vi "FPGA.vi"() -> ()   [LabVIEW 2014]
uses:
  SPI v2/ADXL345 Output.ctl
  <userlib>/_NI SPI IP/FPGA/Controllers/Public/Transfer Settings.ctl
  SPI v2/ADXL345 SPI Statechart.lvsc/Outputs.ctl
  <vilib>/Platform/TimedLoop/XDataNode/timing_clust.ctl
  <vilib>/Platform/TimedLoop/XDataNode/nitl_modes.ctl
  <vilib>/Platform/TimedLoop/XDataNode/wakeup.ctl
  <userlib>/_NI SPI IP/FPGA/Controllers/Public/Spi Master Inputs.ctl
  SPI v2/ADXL345 SPI Statechart.lvsc/Inputs.ctl
  <vilib>/rvi/Emulation/niFpgaGetClockAttributes.vi
  <vilib>/rvi/Emulation/niFpgaSctlEmulationGetInTimedLoop.vi
  <vilib>/rvi/Emulation/niFpgaEmulationReportErrorSimple.vi
  <vilib>/rvi/eio/common/nirviEmuTemplateMethod_errors.vi
  FPGA Globals.vi
  <vilib>/rvi/Emulation/niFpgaCriticalErrorInLSC.vi
  <vilib>/rvi/Emulation/niFpgaProcessEmulError.vi
  SPI v2/ADXL345 SPI Statechart.lvsc/CompanionDiagram.vi/7/SC Main.vi
  <vilib>/eio/EIONode/EIONode.xnode
  <vilib>/rvi/Analysis/measure/butterworth/XNode/niFpgaButterworthFilter.xnode
  <vilib>/Platform/TimedLoop/XDataNode/XDataNode.xnode
  SPI v2/ADXL345 SPI Statechart.lvsc/Trigger.ctl
  <vilib>/Statechart/Infrastructure/RTStatechart/RunTime SCN.xnode
  SPI v2/ADXL345 SPI Statechart.lvsc
  <vilib>/Platform/TimedLoop/XDataNode/XDNodeRunTimeDep.lvlib
  <userlib>/_NI SPI IP/FPGA/Controllers/NI SPI IP FPGA.lvlib
panel:
  in  "bDCDCDisable":bool
  in  "bLapBeaconPickupEnable":bool
  in  "bWheelSpeedsEnable":bool
  in  "bAccumulatorFansEnable":bool
  out "bLapBeaconPickup":bool
  out "tLapDelta":u32
  in  "bResetFastestLap":bool
  out "tFastestLap":u32
  in  "tLapReference":u32
  in  "bWheelFRFail":bool
  in  "bWheelFLFail":bool
  out "ADXL345 Output":T1
  out "rSlipFR":fxp<+/-,12,1>
  out "rSlipFL":fxp<+/-,12,1>
  out "rSlipRR":fxp<+/-,12,1>
  out "rSlipRL":fxp<+/-,12,1>
  out "sLap":fxp<+,32,12>
  out "vCar":fxp<+/-,33,19>
  out "vAxleF":fxp<+/-,33,19>
  in  "bAccel":bool
  out "vWheelHighest":fxp<+/-,32,18>
  out "vWheelLowest":fxp<+/-,32,18>
  out "vWheelFL":fxp<+/-,32,18>
  out "vWheelFR":fxp<+/-,32,18>
  out "vWheelRL":fxp<+/-,32,18>
  out "vWheelRR":fxp<+/-,32,18>
  in  "Tire Diameter(m)":fxp<+,16,1>
  out "nWheelRR":fxp<+/-,29,16>
  out "nWheelRL":fxp<+/-,29,16>
  out "nWheelFR":fxp<+/-,29,16>
  out "nWheelFL":fxp<+/-,29,16>
  out "NLap":u8
  in  "bResetNLap":bool
  out "aSteerWheel":fxp<+/-,22,10>=124.904541015625
  in  "VSteerWheelMiddle":fxp<+/-,26,5>=0.34827280044555664
  out "bBrakeFOK":bool
  out "bBrakeROK":bool
  out "bLowCurrentOK":bool
  out "bHighCurrentOK":bool
  out "pBrakeF":fxp<+,26,13>
  out "pBrakeR":fxp<+,26,13>
  out "ILowCurrent":fxp<+/-,24,15>=4.353515625
  out "IHighCurrent":fxp<+/-,24,15>=-20.724609375
  out "VShockFL":fxp<+/-,24,5>=0.3892974853515625
  out "VShockFR":fxp<+/-,24,5>=0.3425788879394531
  out "VShockRL":fxp<+/-,24,5>=0.3444976806640625
  out "VShockRR":fxp<+/-,24,5>=0.3793773651123047
  in  "bBrakeLight":bool=TRUE
  out "tWheelFLPeriod":u32
  out "tWheelFRPeriod":u32
  out "tWheelRRPeriod":u32
  out "tWheelRLPeriod":u32
  out "bWheelFLStopped":bool=TRUE
  out "bWheelFRStopped":bool=TRUE
  out "bWheelRLStopped":bool=TRUE
  out "bWheelRRStopped":bool=TRUE
  out "VBrakePressureF":fxp<+/-,24,5>=0.4808177947998047
  out "VBrakePressureR":fxp<+/-,24,5>=0.4820976257324219
  out "bWheelFL":bool
  out "bWheelFR":bool
  out "bWheelRR":bool
  out "bWheelRL":bool
  out "V5VSupply":fxp<+/-,24,5>
  in  "tLapMin":u32=15000
  out "tLastLap":u32
  out "bNewLap":bool
  out "tCurrentLap":u32
  in  "bMotorControllerEnable":bool
  out "bTSMSOutStatus":bool
  in  "bSBRIOOK1":bool
  in  "bSBRIOOK2":bool
  out "bBSPDOK":bool
  out "bIMDOK":bool
  out "bBMSOK":bool
  in  "bPosAIREnable":bool
  out "bTSMSInStatus":bool
  in  "bRTDSEnable":bool
  in  "bCoolantPumpEnable":bool
  in  "rTPS1Min":fxp<+,16,4>=0.41015625
  in  "rTPS1Max":fxp<+,16,4>=0.6201171875
  in  "rTPS2Min":fxp<+,16,4>=0.489990234375
  in  "rTPS2Max":fxp<+,16,4>=0.27001953125
  out "rTPS1":fxp<+/-,31,22>
  out "VTPS1":fxp<+/-,24,5>=3.619058609008789
  out "rTPS2":fxp<+/-,31,22>
  out "VTPS2":fxp<+/-,24,5>=1.0001773834228516
  out "rThrottle":fxp<+/-,33,22>
  out "bTPSInRange":bool
  out "bTPSConsistent":bool
  out "rTPS1Unscaled":fxp<+/-,16,1>
  out "rTPS2Unscaled":fxp<+/-,16,1>
  out "TSBRIO":fxp<+,19,8>=27.25 format="%.10g"
  out "bFPGALED":bool
  out "VsbRIOSupply":fxp<+/-,25,6>=13.101043701171875
  in  "VSupplyOffset":fxp<+,12,4>=8.890625
  in  "stop":bool
  out "Tick Count(mSec)":u32
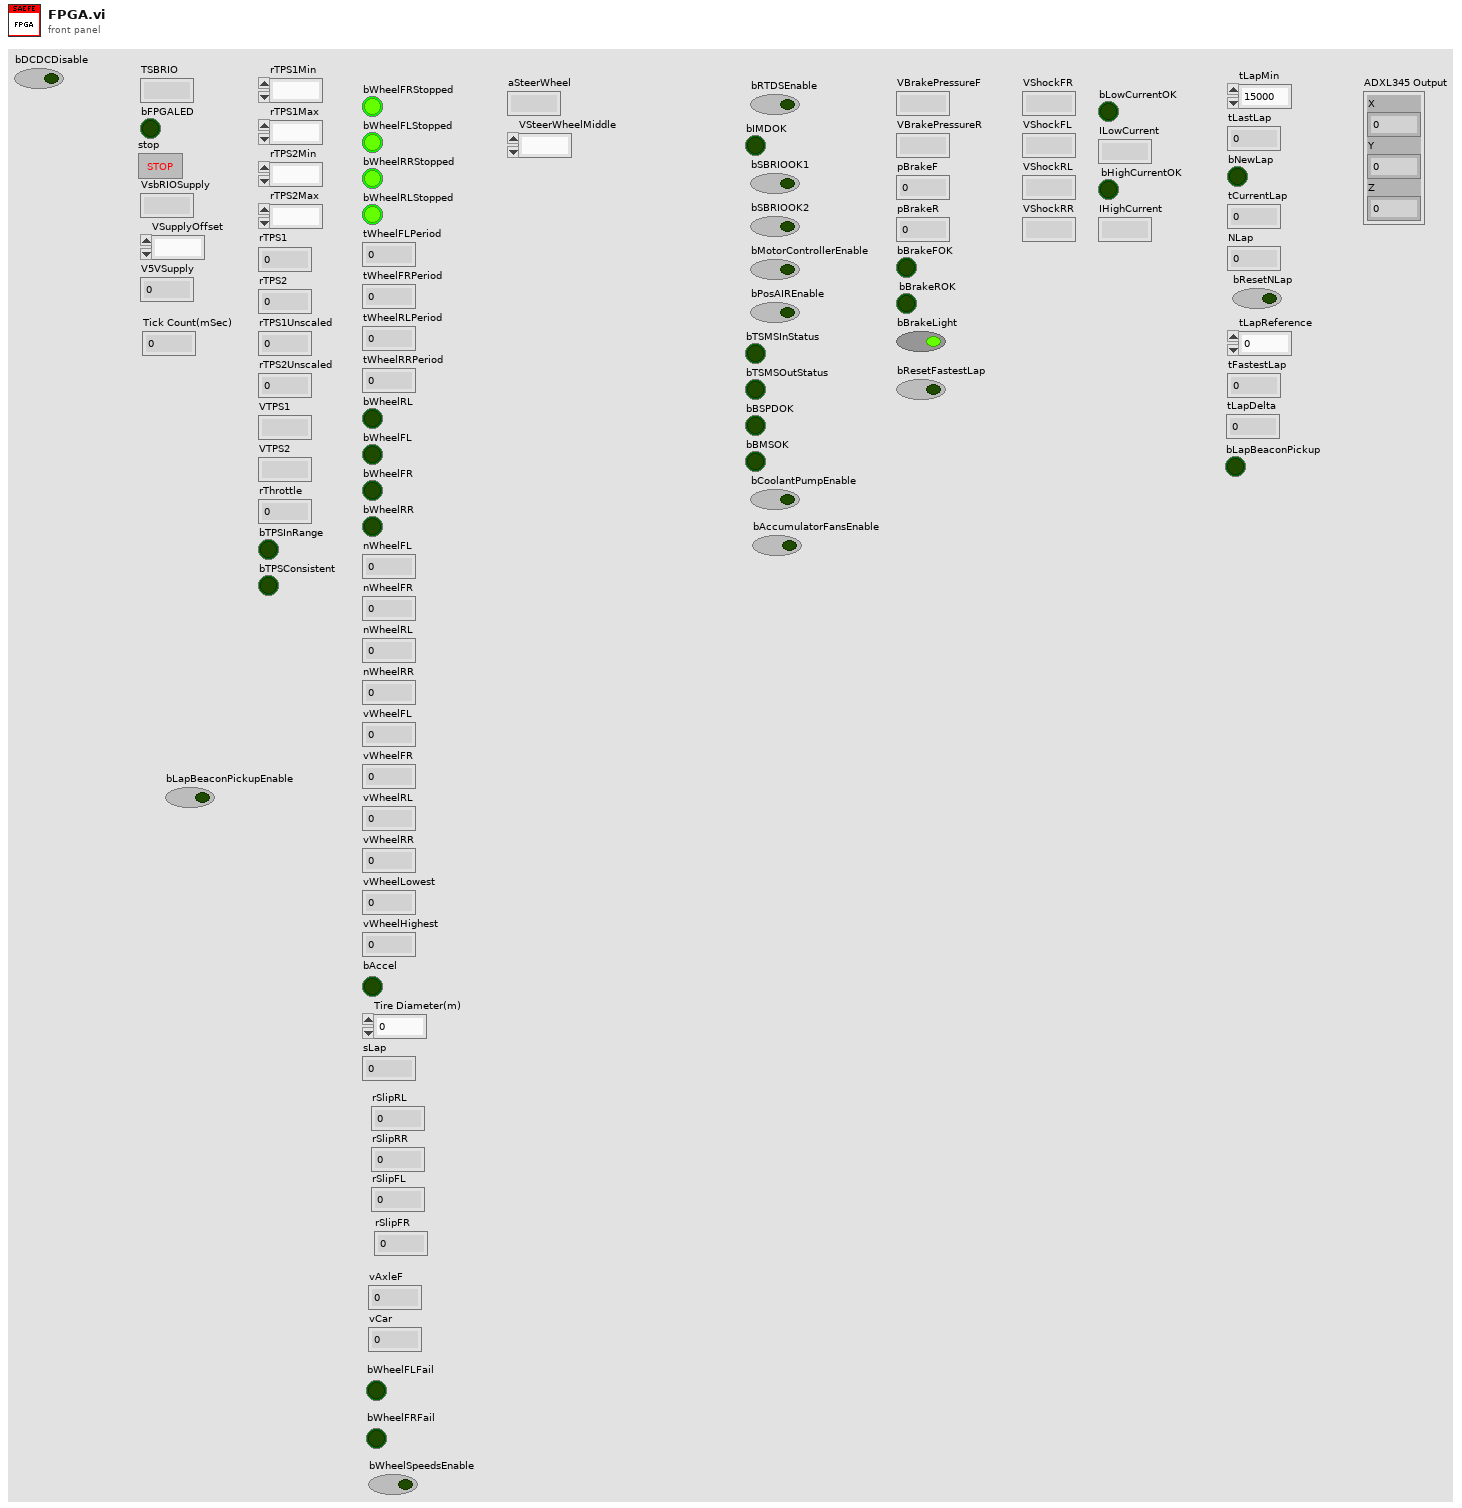
[diagram p1: front panel]
types:
  T1 = typedef "ADXL345 Output.ctl" = cluster{"X":fxp<+/-,14,4>, "Y":fxp<+/-,14,4>, "Z":fxp<+/-,14,4>}
  T2 = typedef "ADXL345 SPI Statechart.lvsc/Outputs.ctl" = cluster{"Transfer Length (bits)":u8, "start strobe":bool, "data to write":u64, "ADXL345 Output":T1}
  T3 = typedef "NI SPI IP FPGA.lvlib/Transfer Settings.ctl" = cluster{"Divide Value":u8, "Transfer Length (bits)":u8, "CS Asserted Polarity":bool, "Clock Polarity (CPOL)":bool, "Clock Phase (CPHA)":bool, "Lengthen MISO Setup":bool, "Direction Change Bit":u8, "MOSI Starts as Output":bool, "Tristatable MOSI":bool}
  T4 = typedef "ADXL345 SPI Statechart.lvsc/Inputs.ctl" = cluster{"read data valid":bool, "read data":u64, "ready for input":bool}
  T5 = typedef "NI SPI IP FPGA.lvlib/Spi Master Inputs.ctl" = cluster{"MISO":bool}
  T6 = typedef "XDNodeRunTimeDep.lvlib/timing_clust.ctl" = cluster{"Expected End [f-1]":u64, "Actual End [f-1]":u64, "Finished Late? [f-1]":bool, "Expected End [i-1]":u64, "Actual End [i-1]":u64, "Finished Late? [i-1]":bool, "Expected Start [i]":u64, "Actual Start [i]":u64, "Expected Start [f]":u64, "Actual Start [f]":u64, "Source Name":string, "Structure Name":string, "Period":i64, "Deadline":i64, "Offset":i64, "Start":i64, "Priority":i32, "Timeout":i32, "Mode":T7, "Wakeup Reason":T8, "Error":errorcluster, "Source Type":string, "Secondary Source Type":string, "Global End Time":u64, "Global Start Time":u64, "Frame Duration":u64, "Iteration Duration":u64, "Assigned CPU":i32, "I/O Scan Engine Mode":u32}
  T7 = typedef "XDNodeRunTimeDep.lvlib/nitl_modes.ctl" = enum32{"No Change", "Process missed periods, maintain original phase", "Discard missed periods, maintain original phase", "Process missed periods, ignore original phase", "Discard missed periods, ignore original phase"}
  T8 = typedef "XDNodeRunTimeDep.lvlib/wakeup.ctl" = enum32{"Normal", "Aborted", "Asynchronous wakeup", "Timing source error", "Timed loop error", "Timeout"}
  T9 = typedef "NI SPI IP FPGA.lvlib/Spi Master Outputs.ctl" = cluster{"Chip Select":bool, "Clock":bool, "MOSI":bool, "MOSI OE":bool}
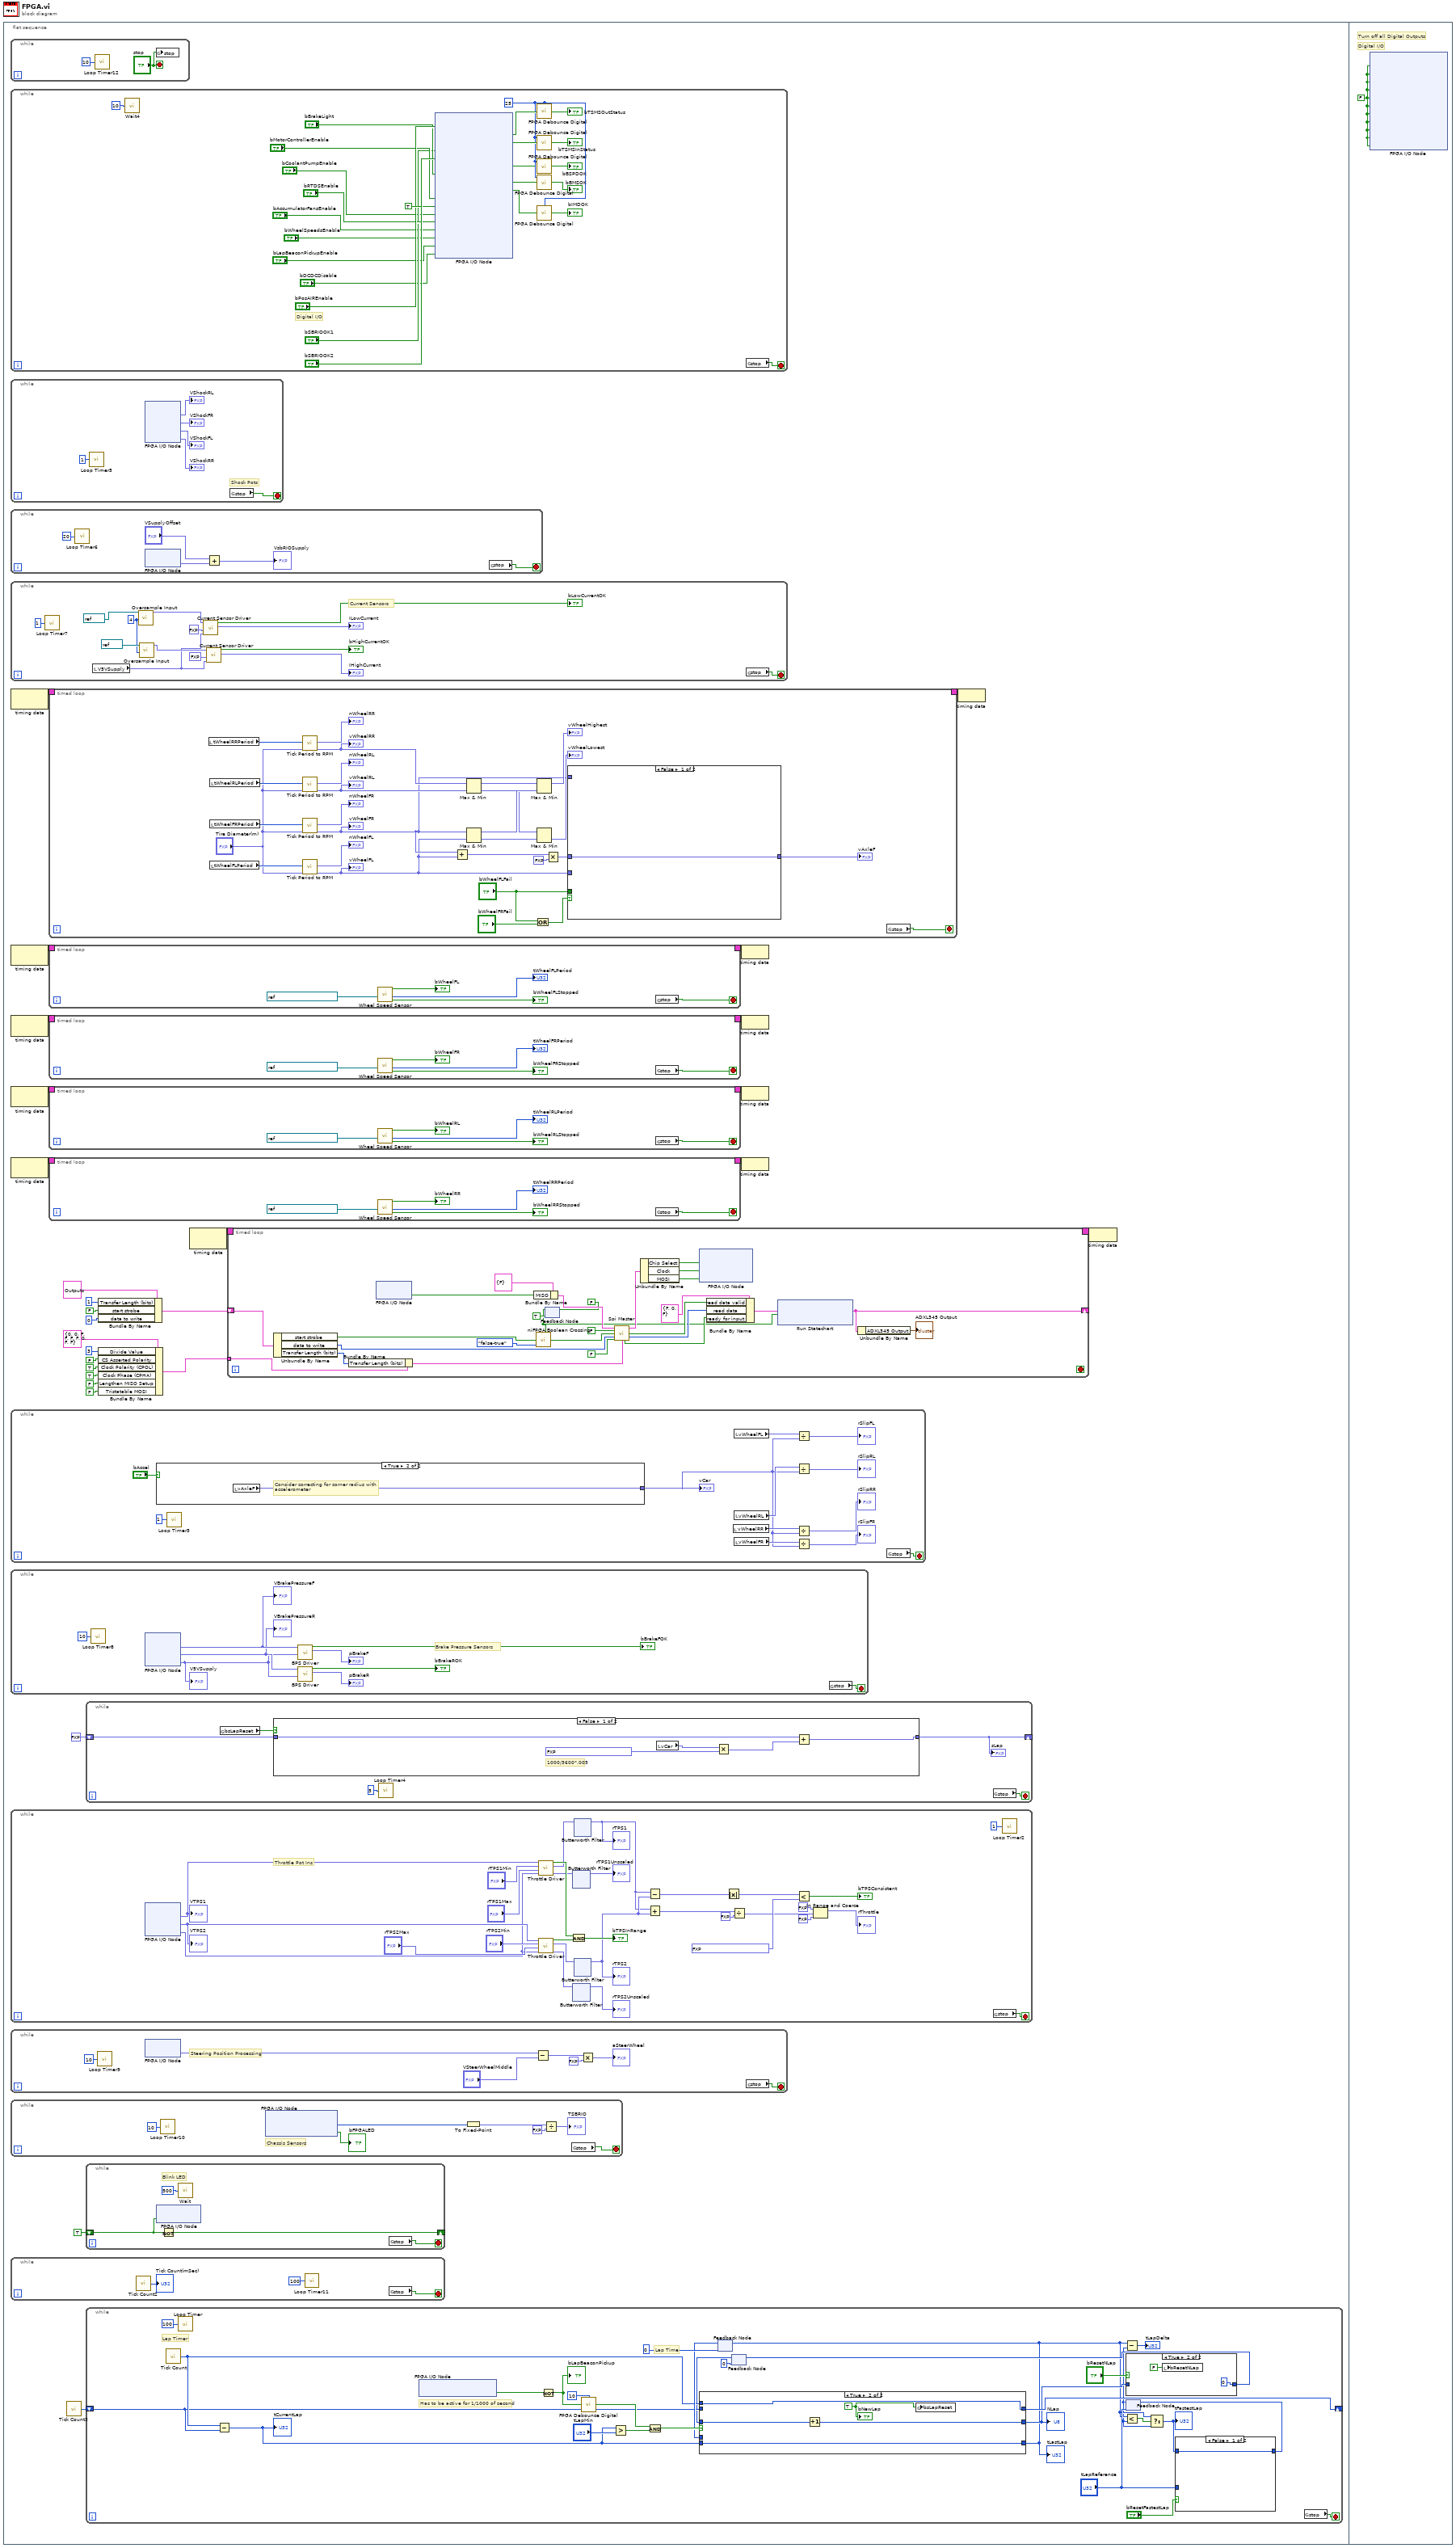
[diagram p0: block diagram]
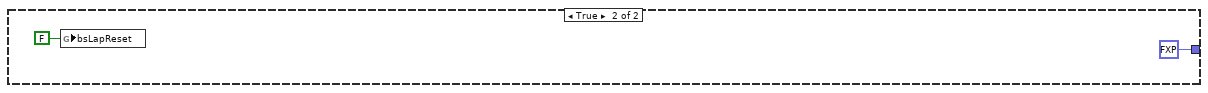
[diagram p2: hidden frame]
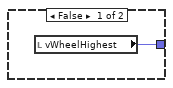
[diagram p3: hidden frame]
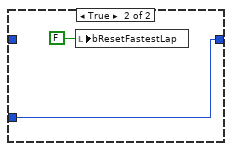
[diagram p6: hidden frame]
diagram:
  n1 = flat-sequence {
    frame #0 {
      n2 = while {
        stop <- "stop" stop-if-true
        n3 = call "Loop Timer12"("Count(mSec)"=u32 10) -> ()  [unwired: 1 out]
        n4 = global write "FPGA Globals.vi" "stop"("stop") -> ()
      }
      n5 = while {
        stop <- w340 stop-if-true
        w330 = u16 25 ("Cycles to Filter")
        # "Digital I/O"
        n6 = call "Wait4"("Count(mSec)"=u32 10) -> ()  [unwired: 1 out]
        n7 = xnode "FPGA I/O Node"("RMC Connector/DIO8"="bPosAIREnable", "RMC Connector/DIO6"="bSBRIOOK1", "RMC Connector/DIO5"="bSBRIOOK2", "RMC Connector/DIO11"="bBrakeLight", "RMC Connector/DIO33"="bMotorControllerEnable", "RMC Connector/DIO14"=TRUE, "RMC Connector/DIO41"="bCoolantPumpEnable", "RMC Connector/DIO40"="bRTDSEnable", "RMC Connector/DIO9"="bAccumulatorFansEnable", "RMC Connector/DIO83"="bWheelSpeedsEnable", "RMC Connector/DIO4"="bLapBeaconPickupEnable", "RMC Connector/DIO45"="bDCDCDisable") -> ("RMC Connector/DIO7"=w338:bool, "RMC Connector/DIO39"=w336:bool, "RMC Connector/DIO1"=w324:bool, "RMC Connector/DIO94"=w323:bool, "RMC Connector/DIO95"=w332:bool)  [unwired: 17 in, 17 out]
        n8 = call "FPGA Debounce Digital.vi"("Input Signal"=w338, "Cycles to Filter"=w330) -> ("Output Filtered Signal"=→"bTSMSOutStatus":bool)
        n9 = call "FPGA Debounce Digital.vi"("Input Signal"=w336, "Cycles to Filter"=w330) -> ("Output Filtered Signal"=→"bTSMSInStatus":bool)
        n10 = call "FPGA Debounce Digital.vi"("Input Signal"=w324, "Cycles to Filter"=w330) -> ("Output Filtered Signal"=→"bBSPDOK":bool)
        n11 = call "FPGA Debounce Digital.vi"("Input Signal"=w323, "Cycles to Filter"=w330) -> ("Output Filtered Signal"=→"bBMSOK":bool)
        n12 = call "FPGA Debounce Digital.vi"("Input Signal"=w332, "Cycles to Filter"=w330) -> ("Output Filtered Signal"=→"bIMDOK":bool)
        n13 = global read "FPGA Globals.vi" "stop"() -> (w340:bool)
      }
      n14 = while {
        stop <- w229 stop-if-true
        # "Shock Pots"
        n15 = call "Loop Timer5"("Count(mSec)"=u32 1) -> ()  [unwired: 1 out]
        n16 = xnode "FPGA I/O Node"() -> ("AI9"=→"VShockRL":fxp<+/-,24,5>, "AI10"=→"VShockFR":fxp<+/-,24,5>, "AI11"=→"VShockFL":fxp<+/-,24,5>, "AI8"=→"VShockRR":fxp<+/-,24,5>)  [unwired: 4 in, 4 out]
        n17 = global read "FPGA Globals.vi" "stop"() -> (w229:bool)
      }
      n18 = while {
        stop <- w213 stop-if-true
        n19 = call "Loop Timer6"("Count(mSec)"=u32 20) -> ()  [unwired: 1 out]
        n20 = xnode "FPGA I/O Node"() -> ("AI0"=w216:fxp<+/-,24,5>)  [unwired: 1 in, 1 out]
        n21 = Add(x="VSupplyOffset", y=w216) -> (x+y=→"VsbRIOSupply":fxp<+/-,25,6>)
        n22 = global read "FPGA Globals.vi" "stop"() -> (w213:bool)
      }
      n23 = while {
        stop <- w240 stop-if-true
        w237 = u8 4 ("NSamples")
        # "Current Sensors"
        n24 = call "Loop Timer7"("Count(mSec)"=u32 1) -> ()  [unwired: 1 out]
        n25 = local read "V5VSupply"() -> (w235:fxp<+/-,24,5>)
        n26 = call "Oversample Input.vi"("NSamples"=w237, "Channel"=refnum<k21> "AI2" ("FPGA I/O In")) -> ("Output"=w246:fxp<+/-,36,9>)  [unwired: 9 in]
        n27 = call "Oversample Input.vi"("NSamples"=w237, "Channel"=refnum<k21> "AI1") -> ("Output"=w236:fxp<+/-,36,9>)  [unwired: 9 in]
        n28 = call "Current Sensor Driver.vi"("VSupply"=w235, "IRange"=fxp<+,27,10> 50.0 ("Range"), "VInput"=w246) -> ("ISensor"=→"ILowCurrent":fxp<+/-,24,15>, "bSensorOK"=→"bLowCurrentOK":bool)  [unwired: 7 in]
        n29 = call "Current Sensor Driver.vi"("VSupply"=w235, "IRange"=fxp<+,27,10> 600.0 ("Range"), "VInput"=w236) -> ("ISensor"=→"IHighCurrent":fxp<+/-,24,15>, "bSensorOK"=→"bHighCurrentOK":bool)  [unwired: 7 in]
        n30 = global read "FPGA Globals.vi" "stop"() -> (w240:bool)
      }
      n31 = node-c288() -> (w18:T6)  [unwired: 1 in]
      n32 = node-c288() -> (w27:T6)  [unwired: 1 in]
      n33 = node-c288() -> (w25:T6)  [unwired: 1 in]
      n34 = node-c288() -> (w23:T6)  [unwired: 1 in]
      n35 = node-c288() -> (w21:T6)  [unwired: 1 in]
      n36 = while {
        stop <- w88 stop-if-true
        n37 = case shown="True" "bAccel" {
          tunnel: [w89 w90] -> w78
          frame False {
            n38 = local read "vWheelHighest"() -> (w89:fxp<+/-,32,18>)
          }
          frame True {
            # "Consider correcting for corner radius with\naccelerometer"
            n39 = local read "vAxleF"() -> (w90:fxp<+/-,33,19>)
          }
        }
        "vCar" <- w78
        n40 = call "Loop Timer3"("Count(mSec)"=u32 1) -> ()  [unwired: 1 out]
        n41 = local read "vWheelRR"() -> (w83:fxp<+/-,32,18>)
        n42 = local read "vWheelFL"() -> (w81:fxp<+/-,32,18>)
        n43 = local read "vWheelRL"() -> (w85:fxp<+/-,32,18>)
        n44 = local read "vWheelFR"() -> (w79:fxp<+/-,32,18>)
        n45 = Divide(x=w81, y=w78) -> (x/y=→"rSlipFL":fxp<+/-,12,1>)
        n46 = Divide(x=w85, y=w78) -> (x/y=→"rSlipRL":fxp<+/-,12,1>)
        n47 = Divide(x=w83, y=w78) -> (x/y=→"rSlipRR":fxp<+/-,12,1>)
        n48 = Divide(x=w79, y=w78) -> (x/y=→"rSlipFR":fxp<+/-,12,1>)
        n49 = global read "FPGA Globals.vi" "stop"() -> (w88:bool)
      }
      n50 = while {
        stop <- w250 stop-if-true
        # "Brake Pressure Sensors"
        n51 = call "Loop Timer8"("Count(mSec)"=u32 10) -> ()  [unwired: 1 out]
        n52 = xnode "FPGA I/O Node"() -> ("AI3"=w255:fxp<+/-,24,5>, "AI4"=w253:fxp<+/-,24,5>, "AI14"=w249:fxp<+/-,24,5>)  [unwired: 3 in, 3 out]
        "VBrakePressureF" <- w255
        "VBrakePressureR" <- w253
        "V5VSupply" <- w249
        n53 = call "BPS Driver.vi"("Supply Voltage"=w249, "Signal In"=w255) -> ("Brake Pressure (psi)"=→"pBrakeF":fxp<+,26,13>, "Sensor OK?"=→"bBrakeFOK":bool)  [unwired: 8 in]
        n54 = call "BPS Driver.vi"("Supply Voltage"=w249, "Signal In"=w253) -> ("Brake Pressure (psi)"=→"pBrakeR":fxp<+,26,13>, "Sensor OK?"=→"bBrakeROK":bool)  [unwired: 8 in]
        n55 = global read "FPGA Globals.vi" "stop"() -> (w250:bool)
      }
      n56 = while {
        stop <- w274 stop-if-true
        # "Throttle Pot Ins"
        n57 = xnode "FPGA I/O Node"() -> ("AI5"=w267:fxp<+/-,24,5>, "AI6"=w277:fxp<+/-,24,5>, "AI14"=w271:fxp<+/-,24,5>)  [unwired: 3 in, 3 out]
        "VTPS1" <- w267
        "VTPS2" <- w277
        n58 = call "Throttle Driver.vi"("Reference Voltage In"=w271, "Throttle Max"="rTPS1Max", "Throttle Min"="rTPS1Min", "Throttle Voltage In"=w267) -> ("Unscaled Throttle Percent"=w266:fxp<+/-,16,1>, "Throttle Percent"=w259:fxp<+/-,27,18>, "In Range"=w280:bool)  [unwired: 5 in]
        n59 = call "Throttle Driver.vi"("Reference Voltage In"=w271, "Throttle Max"="rTPS2Max", "Throttle Min"="rTPS2Min", "Throttle Voltage In"=w277) -> ("Unscaled Throttle Percent"=w264:fxp<+/-,16,1>, "Throttle Percent"=w262:fxp<+/-,27,18>, "In Range"=w279:bool)  [unwired: 5 in]
        n60 = xnode "Butterworth Filter"("input data"=w266) -> ("output data"=→"rTPS1Unscaled":fxp<+/-,16,1>)  [unwired: 2 in]
        n61 = xnode "Butterworth Filter"("input data"=w264) -> ("output data"=→"rTPS2Unscaled":fxp<+/-,16,1>)  [unwired: 2 in]
        n62 = Compound Arithmetic op=AND(w280, w279) -> (→"bTPSInRange":bool)
        n63 = xnode "Butterworth Filter"("input data"=w259) -> ("output data"=w258:fxp<+/-,31,22>)  [unwired: 2 in]
        "rTPS1" <- w258
        n64 = xnode "Butterworth Filter"("input data"=w262) -> ("output data"=w261:fxp<+/-,31,22>)  [unwired: 2 in]
        "rTPS2" <- w261
        n65 = Subtract(x=w258, y=w261) -> (x-y=w273:fxp<+/-,32,23>)
        n66 = Add(x=w258, y=w261) -> (x+y=w282:fxp<+/-,32,23>)
        n67 = Absolute Value(x=w273) -> (abs(x)=w272:fxp<+,31,22>)
        n68 = Divide(x=w282, y=fxp<+,1,2> 2.0) -> (x/y=w260:fxp<+/-,33,22>)
        n69 = Less?(x=w272, y=fxp<+/-,46,20> 0.09999999403953552) -> (x < y?=→"bTPSConsistent":bool)
        n70 = In Range and Coerce(upper limit=fxp<+/-,33,22> 1.0, x=w260, lower limit=fxp<+/-,33,22> 0.0) -> (coerced(x)=→"rThrottle":fxp<+/-,33,22>)  [unwired: 1 out]
        n71 = global read "FPGA Globals.vi" "stop"() -> (w274:bool)
        n72 = call "Loop Timer2"("Count(mSec)"=u32 1) -> ()  [unwired: 1 out]
      }
      n73 = while {
        stop <- w343 stop-if-true
        # "Steering Position Processing"
        n74 = call "Loop Timer9"("Count(mSec)"=u32 10) -> ()  [unwired: 1 out]
        n75 = xnode "FPGA I/O Node"() -> ("AI14"=w348:fxp<+/-,24,5>)  [unwired: 1 in, 1 out]
        n76 = Subtract(x=w348, y="VSteerWheelMiddle") -> (x-y=w346:fxp<+/-,27,6>)
        n77 = Multiply(x=w346, y=fxp<+,4,7> 72.0) -> (x*y=→"aSteerWheel":fxp<+/-,22,10>)
        n78 = global read "FPGA Globals.vi" "stop"() -> (w343:bool)
      }
      n79 = while {
        stop <- w222 stop-if-true
        # "Chassis Sensors"
        n80 = call "Loop Timer10"("Count(mSec)"=u32 10) -> ()  [unwired: 1 out]
        n81 = xnode "FPGA I/O Node"() -> ("Chassis Temperature"=w224:i16, "FPGA LED"=→"bFPGALED":bool)  [unwired: 2 in, 2 out]
        n82 = To Fixed-Point(number=w224) -> (fixed-point=w225:fxp<+/-,16,9>)  [unwired: 1 in]
        n83 = Divide(x=w225, y=fxp<+/-,16,9> 4.0) -> (x/y=→"TSBRIO":fxp<+,19,8>)
        n84 = global read "FPGA Globals.vi" "stop"() -> (w222:bool)
      }
      n85 = while {
        stop <- w208 stop-if-true
        n86 = call "Tick Count2"() -> ("Tick Count(mSec)"=→"Tick Count(mSec)":u32)
        n87 = call "Loop Timer11"("Count(uSec)"=u32 100) -> ()  [unwired: 1 out]
        n88 = global read "FPGA Globals.vi" "stop"() -> (w208:bool)
      }
      n89 = timed-loop {
        timing: w18 -> [_]
        timing-out: [_] -> w17
        stop <- w110 stop-if-true
        n90 = local read "tWheelRRPeriod"() -> (w111:u32)
        n91 = local read "tWheelRLPeriod"() -> (w112:u32)
        n92 = local read "tWheelFRPeriod"() -> (w113:u32)
        n93 = local read "tWheelFLPeriod"() -> (w114:u32)
        n94 = call "Tick Period to RPM.vi"("Tire Diameter(m)"="Tire Diameter(m)", "Tick Period"=w111) -> ("vWheel"=w107:fxp<+/-,32,18>, "nWheel"=→"nWheelRR":fxp<+/-,29,16>)  [unwired: 8 in]
        "vWheelRR" <- w107
        n95 = call "Tick Period to RPM.vi"("Tire Diameter(m)"="Tire Diameter(m)", "Tick Period"=w112) -> ("vWheel"=w106:fxp<+/-,32,18>, "nWheel"=→"nWheelRL":fxp<+/-,29,16>)  [unwired: 8 in]
        "vWheelRL" <- w106
        n96 = call "Tick Period to RPM.vi"("Tire Diameter(m)"="Tire Diameter(m)", "Tick Period"=w113) -> ("vWheel"=w93:fxp<+/-,32,18>, "nWheel"=→"nWheelFR":fxp<+/-,29,16>)  [unwired: 8 in]
        "vWheelFR" <- w93
        n97 = call "Tick Period to RPM.vi"("Tire Diameter(m)"="Tire Diameter(m)", "Tick Period"=w114) -> ("vWheel"=w92:fxp<+/-,32,18>, "nWheel"=→"nWheelFL":fxp<+/-,29,16>)  [unwired: 8 in]
        "vWheelFL" <- w92
        n98 = Add(x=w93, y=w92) -> (x+y=w99:fxp<+/-,33,19>)
        n99 = Max & Min(x=w107, y=w106) -> (max(x,y)=w104:fxp<+/-,32,18>, min(x,y)=w103:fxp<+/-,32,18>)
        n100 = Max & Min(x=w93, y=w92) -> (max(x,y)=w105:fxp<+/-,32,18>, min(x,y)=w102:fxp<+/-,32,18>)
        n101 = Or(x="bWheelFLFail", y="bWheelFRFail") -> (x .or. y?=w91:bool)
        n102 = Max & Min(x=w104, y=w105) -> (max(x,y)=→"vWheelHighest":fxp<+/-,32,18>)  [unwired: 1 out]
        n103 = Max & Min(x=w103, y=w102) -> (min(x,y)=→"vWheelLowest":fxp<+/-,32,18>)  [unwired: 1 out]
        n104 = Multiply(x=w99, y=fxp<+/-,33,19> 0.5) -> (x*y=w96:fxp<+/-,33,19>)
        n105 = case shown="False" w91 {
          tunnel: w96 -> [w118 _]
          tunnel: [w118 w120] -> w95
          tunnel: "bWheelFLFail" -> [_ w122]
          tunnel: w93 -> [_ w121]
          tunnel: w92 -> [_ w119]
          frame False {
          }
          frame True {
            n106 = case shown="False" w122 {
              tunnel: w121 -> [_ w124]
              tunnel: [w123 w124] -> w120
              tunnel: w119 -> [w123 _]
              frame False {
              }
              frame True {
              }
            }
          }
        }
        "vAxleF" <- w95
        n107 = global read "FPGA Globals.vi" "stop"() -> (w110:bool)
      }
      n108 = timed-loop {
        timing: w27 -> [_]
        timing-out: [_] -> w26
        stop <- w198 stop-if-true
        n109 = call "Wheel Speed Sensor.vi"("FPGA I/O In"=refnum<k21> "RMC Connector/DIO88") -> ("Stopped"=→"bWheelFLStopped":bool, "Tick Period"=→"tWheelFLPeriod":u32, "State Out"=→"bWheelFL":bool)  [unwired: 8 in]
        n110 = global read "FPGA Globals.vi" "stop"() -> (w198:bool)
      }
      n111 = timed-loop {
        timing: w25 -> [_]
        timing-out: [_] -> w24
        stop <- w190 stop-if-true
        n112 = call "Wheel Speed Sensor.vi"("FPGA I/O In"=refnum<k21> "RMC Connector/DIO87") -> ("Stopped"=→"bWheelFRStopped":bool, "Tick Period"=→"tWheelFRPeriod":u32, "State Out"=→"bWheelFR":bool)  [unwired: 8 in]
        n113 = global read "FPGA Globals.vi" "stop"() -> (w190:bool)
      }
      n114 = timed-loop {
        timing: w23 -> [_]
        timing-out: [_] -> w22
        stop <- w181 stop-if-true
        n115 = call "Wheel Speed Sensor.vi"("FPGA I/O In"=refnum<k21> "RMC Connector/DIO86") -> ("Stopped"=→"bWheelRLStopped":bool, "Tick Period"=→"tWheelRLPeriod":u32, "State Out"=→"bWheelRL":bool)  [unwired: 8 in]
        n116 = global read "FPGA Globals.vi" "stop"() -> (w181:bool)
      }
      n117 = timed-loop {
        timing: w21 -> [_]
        timing-out: [_] -> w20
        stop <- w172 stop-if-true
        n118 = call "Wheel Speed Sensor.vi"("FPGA I/O In"=refnum<k21> "RMC Connector/DIO85") -> ("Stopped"=→"bWheelRRStopped":bool, "Tick Period"=→"tWheelRRPeriod":u32, "State Out"=→"bWheelRR":bool)  [unwired: 8 in]
        n119 = global read "FPGA Globals.vi" "stop"() -> (w172:bool)
      }
      n120 = call "Tick Count3"() -> ("Tick Count(mSec)"=w19:u32)
      n121 = while {
        shift-right: [w65] -> _
        shift-left: fxp<+,32,12> 0.0 -> [w66]
        stop <- w69 stop-if-true
        n122 = global read "FPGA Globals.vi" "bsLapReset"() -> (w67:bool)
        n123 = case shown="False" w67 {
          tunnel: w66 -> [w71 _]
          tunnel: [w70 fxp<+,32,12> 0.0] -> w65
          frame False {
            # "1000/3600*.005"
            n124 = local read "vCar"() -> (w74:fxp<+/-,33,19>)
            n125 = Multiply(x=w74, y=fxp<+,32,4> 0.00138888880610466) -> (x*y=w72:fxp<+,32,12>)
            n126 = Add(x=w71, y=w72) -> (x+y=w70:fxp<+,32,12>)
          }
          frame True {
            n127 = global write "FPGA Globals.vi" "bsLapReset"(FALSE ("bsLapReset")) -> ()
          }
        }
        "sLap" <- w65
        n128 = call "Loop Timer4"("Count(mSec)"=u32 5) -> ()  [unwired: 1 out]
        n129 = global read "FPGA Globals.vi" "stop"() -> (w69:bool)
      }
      n130 = while {
        shift-right: [w218] -> _
        shift-left: TRUE ("FPGA LED") -> [w219]
        stop <- w217 stop-if-true
        # "Blink LED"
        n131 = xnode "FPGA I/O Node"("FPGA LED"=w219) -> ()  [unwired: 1 in, 1 out]
        n132 = Not(x=w219) -> (.not. x?=w218:bool)
        n133 = call "Wait"("Count(mSec)"=u32 500) -> ()  [unwired: 1 out]
        n134 = global read "FPGA Globals.vi" "stop"() -> (w217:bool)
      }
      n135 = while {
        shift-right: [w145] -> _
        shift-left: w19 -> [w144]
        stop <- w154 stop-if-true
        # "Lap Time"
        # "Lap Timer"
        # "Has to be active for 1/1000 of second"
        n136 = call "Tick Count"() -> ("Tick Count(mSec)"=w146:u32)
        n137 = call "Loop Timer"("Count(uSec)"=u32 100) -> ()  [unwired: 1 out]
        n138 = Subtract(x=w146, y=w144) -> (x-y=w149:u32)
        "tCurrentLap" <- w149
        n139 = xnode "FPGA I/O Node"() -> ("RMC Connector/DIO12"=w129:bool)  [unwired: 1 in, 1 out]
        n140 = Not(x=w129) -> (.not. x?=w130:bool)
        "bLapBeaconPickup" <- w130
        n141 = call "FPGA Debounce Digital.vi"("Input Signal"=w130, "Cycles to Filter"=u16 10) -> ("Output Filtered Signal"=w152:bool)
        n142 = Greater?(x=w149, y="tLapMin") -> (0:w151:bool)
        n143 = And(x=w152, y=w151) -> (x .and. y?=w150:bool)
        n144 = feedback #1(u32 0) -> (w147:u32)
        n145 = feedback #2(u8 0) -> (w142:u8)
        n146 = case shown="True" w150 {
          tunnel: w149 -> [_ w170]
          tunnel: [w165 w170] -> w133
          tunnel: w147 -> [w165 _]
          tunnel: w146 -> [_ w169]
          tunnel: [w164 w169] -> w145
          tunnel: w144 -> [w164 _]
          tunnel: w142 -> [w163 w168]
          tunnel: [w163 w167] -> w140
          frame False {
          }
          frame True {
            w166 = TRUE
            n147 = Increment(x=w168) -> (x+1=w167:u8)
            n148 = global write "FPGA Globals.vi" "bsLapReset"(w166) -> ()
            "bNewLap" <- w166
          }
        }
        "tLastLap" <- w133
        "NLap" <- w140
        n149 = feedback-in #1(w133) -> ()
        n150 = case shown="True" "bResetNLap" {
          tunnel: w140 -> [w160 _]
          tunnel: [w160 u8 0] -> w139
          frame False {
          }
          frame True {
            n151 = local write "bResetNLap"(FALSE ("bResetNLap")) -> ()
          }
        }
        n152 = feedback-in #2(w139) -> ()
        n153 = feedback #3("tLapReference") -> (w132:u32)
        n154 = Subtract(x=w133, y=w132) -> (x-y=→"tLapDelta":u32)
        n155 = Less?(x=w133, y=w132) -> (x < y?=w138:bool)
        n156 = Select(t=w133, s=w138, f=w132) -> (s? t:f=w136:u32)
        "tFastestLap" <- w136
        n157 = case shown="False" "bResetFastestLap" {
          tunnel: w136 -> [w157 _]
          tunnel: "tLapReference" -> [_ w158]
          tunnel: [w157 w158] -> w134
          frame False {
          }
          frame True {
            n158 = local write "bResetFastestLap"(FALSE ("bResetFastestLap")) -> ()
          }
        }
        n159 = feedback-in #3(w134) -> ()
        n160 = global read "FPGA Globals.vi" "stop"() -> (w154:bool)
      }
      n161 = Bundle By Name(cluster=T2 {"Transfer Length (bits)"=0, "start strobe"=FALSE, "data to write"=0, "ADXL345 Output"={"X"=0.0, "Y"=0.0, "Z"=0.0}} ("Outputs"), "Transfer Length (bits)"=u8 1, "start strobe"=FALSE, "data to write"=u64 0) -> (w4:T2)
      n162 = Bundle By Name(cluster=T3 {"Divide Value"=0, "Transfer Length (bits)"=0, "CS Asserted Polarity"=FALSE, "Clock Polarity (CPOL)"=FALSE, "Clock Phase (CPHA)"=FALSE, "Lengthen MISO Setup"=FALSE, "Direction Change Bit"=0, "MOSI Starts as Output"=FALSE, "Tristatable MOSI"=FALSE} ("spi transfer settings"), "Divide Value"=u8 3, "CS Asserted Polarity"=FALSE, "Clock Polarity (CPOL)"=TRUE, "Clock Phase (CPHA)"=TRUE, "Lengthen MISO Setup"=FALSE, "Tristatable MOSI"=FALSE) -> (w10:T3)
      n163 = node-c288() -> (w15:T6)  [unwired: 1 in]
      n164 = timed-loop {
        timing: w15 -> [_]
        timing-out: [_] -> w14
        tunnel: w10 -> [w39]
        shift-right: [w30] -> _
        shift-left: w4 -> [w41]
        stop <- _ stop-if-true
        n165 = Unbundle By Name(w41) -> ("start strobe"=w35:bool, "data to write"=w36:u64, "Transfer Length (bits)"=w37:u8)
        n166 = Bundle By Name(cluster=w39, "Transfer Length (bits)"=w37) -> (w38:T3)
        n167 = xnode "FPGA I/O Node"() -> ("MISO"=w54:bool)  [unwired: 1 in, 1 out]
        n168 = Bundle By Name(cluster=T5 {"MISO"=FALSE} ("spi input"), "MISO"=w54) -> (w53:T5)
        n169 = feedback-in #4(FALSE) -> ()
        n170 = feedback #4(TRUE) -> (w32:bool)
        n171 = call <vilib>:"niFPGA Boolean Crossing.vi"("input"=w35, "direction"=enum8{"either", "false-true", "true-false"}."false-true", "initialize"=w32) -> ("crossing"=w34:bool)  [unwired: 6 in]
        n172 = call <userlib>:"Spi Master.vi"("spi input"=w53, "manual assert chip select"=FALSE, "start strobe"=w34, "data to write"=w36, "MOSI output enable done"=FALSE, "spi transfer settings"=w38) -> ("spi output"=w45:T9, "read data valid"=w51:bool, "read data"=w50:u64, "ready for input"=w49:bool)  [unwired: 6 in]
        n173 = Unbundle By Name(w45) -> ("Chip Select"=w44:bool, "Clock"=w43:bool, "MOSI"=w42:bool)
        n174 = xnode "FPGA I/O Node"("ACCEL Select"=w44, "CLK"=w43, "MOSI"=w42) -> ()  [unwired: 3 in, 3 out]
        n175 = Bundle By Name(cluster=T4 {"read data valid"=FALSE, "read data"=0, "ready for input"=FALSE} ("Inputs"), "read data valid"=w51, "read data"=w50, "ready for input"=w49) -> (w48:T4)
        n176 = xnode "Run Statechart"("Init?"=w32, "Inputs"=w48) -> ("Outputs"=w30:T2)  [unwired: 1 in, 1 out]
        n177 = Unbundle By Name(w30) -> ("ADXL345 Output"=→"ADXL345 Output":T1)
      }
      n178 = node-c288(w26) -> ()
      n179 = node-c288(w24) -> ()
      n180 = node-c288(w22) -> ()
      n181 = node-c288(w20) -> ()
      n182 = node-c288(w17) -> ()
      n183 = node-c288(w14) -> ()
    }
    frame #1 {
      w349 = FALSE
      # "Turn off all Digital Outputs"
      # "Digital I/O"
      n184 = xnode "FPGA I/O Node"("RMC Connector/DIO8"=w349, "RMC Connector/DIO6"=w349, "RMC Connector/DIO5"=w349, "RMC Connector/DIO40"=w349, "RMC Connector/DIO40"=w349, "RMC Connector/DIO11"=w349, "RMC Connector/DIO33"=w349, "RMC Connector/DIO14"=w349, "RMC Connector/DIO41"=w349, "RMC Connector/DIO11"=w349, "RMC Connector/DIO9"=w349) -> ()  [unwired: 11 in, 11 out]
    }
  }
